vi "test_Create MetaData Channel_error on empty name.vi"(8 "error in (no error)":errorcluster, 11 "TestCase in":refnum<class "Instrument Addon Scripting API Channels Unit Tests.lvclass">) -> (0 "error out":errorcluster, 3 "TestCase out":refnum<class "Instrument Addon Scripting API Channels Unit Tests.lvclass">)   [LabVIEW 2018, in "Instrument Addon Scripting API Channels Unit Tests.lvclass"]
uses:
  Instrument Addon Scripting API Channels Unit Tests.lvclass
  APIs/Scripting API/TypeDefs/Single Channel Format Settings.ctl
  Instrument Addon Scripting API Channels Unit Tests.lvclass/Instrument Addon Scripting API Channels Unit Tests.ctl
  <vilib>/NI Veristand/Custom Device Tools/Custom Device Utility Library/NI VeriStand - Search for Item by Name.vi
  APIs/Scripting API/Channels/Create MetaData Channel - Single Channel - Format.vi
  <vilib>/addons/_JKI Toolkits/VI Tester/TestCase.llb/TestCase.lvclass
  Instrument Addon Scripting API Test Assets/Instrument Addon Scripting API Test Assets.lvclass
  <vilib>/NI Veristand/Custom Device Tools/Custom Device Utility Library/Custom Device Utility Library.lvlib
  APIs/Scripting API/Instrument Addon Scripting API.lvlib
  C:/Program Files (x86)/National Instruments/LabVIEW 2018/vi.lib/addons/_JKI Toolkits/VI Tester/TestCase.llb/TestCase.lvclass
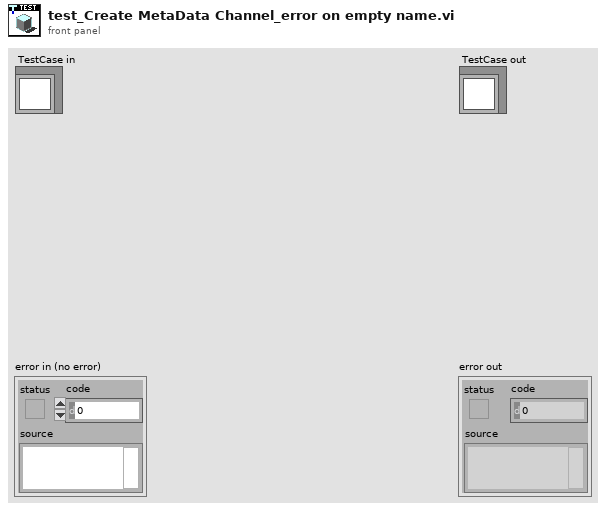
[diagram p1: front panel]
types:
  T1 = typedef "Instrument Addon Scripting API.lvlib/Single Channel Format Settings.ctl" = cluster{"Format String":string, "Default Value":dbl, "Units":string}
  T2 = typedef "Custom Device API.lvlib/Custom Device Item Ref.ctl" = u64
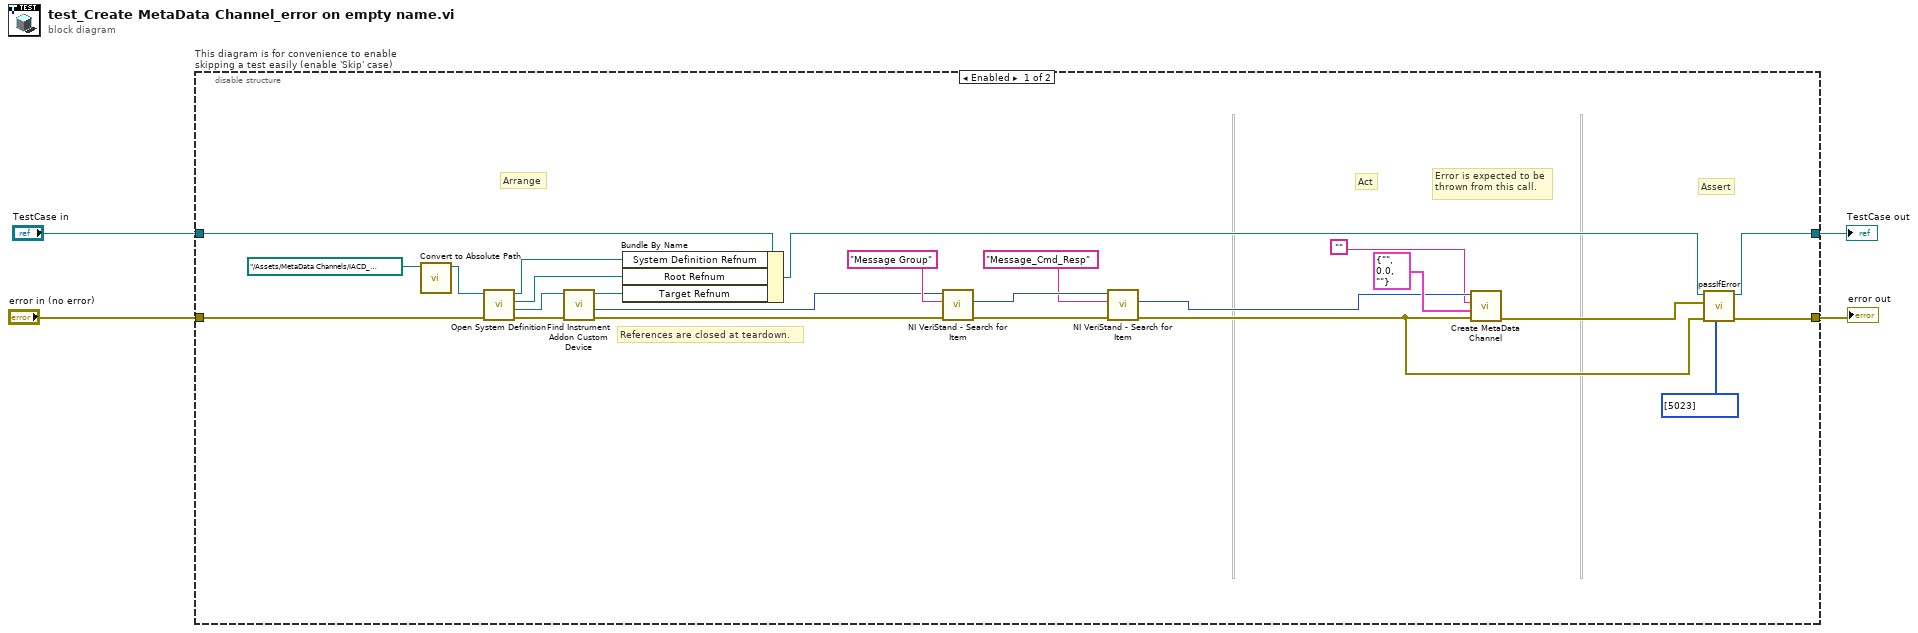
[diagram p0: block diagram]
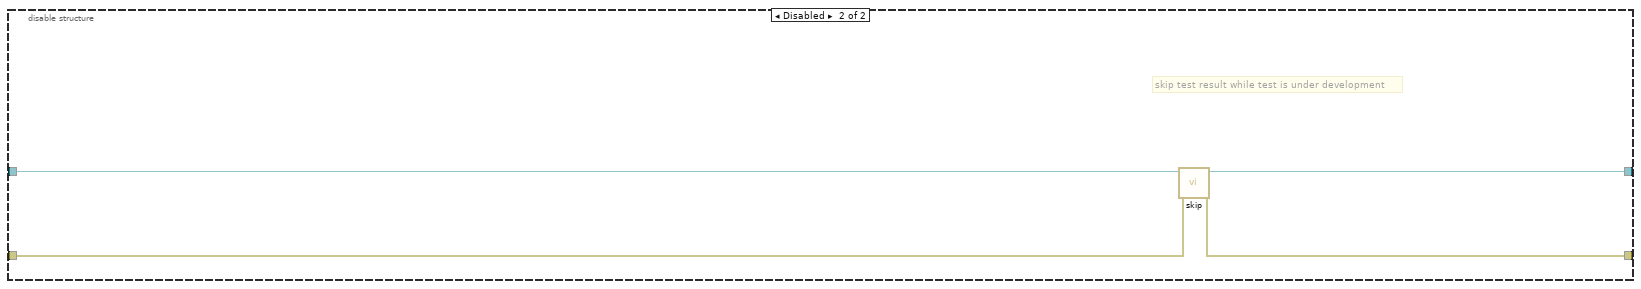
[diagram p2: hidden frame]
diagram:
  n1 = disable-structure "This diagram is for convenience to enable skipping a test easily (enable 'Skip' case)" shown="Enabled" {
    disable-tunnel: "TestCase in" -> [w20 w32]
    disable-tunnel: [w25 w30] -> w1
    disable-tunnel: [w24 w31] -> w3
    disable-tunnel: "error in (no error)" -> [w28 w29]
    frame Enabled {
      # "Error is expected to be\nthrown from this call."
      # "Assert"
      # "References are closed at teardown."
      # "Act"
      # "Arrange"
      n2 = call "Convert to Absolute Path.vi"("System Definition File"=path "../Assets/MetaData Channels/IACD_channels.nivssdf") -> ("Absolute Path"=w5:path)  [unwired: 10 in]
      n3 = call "Open System Definition.vi"("error in (no error)"=w28, "System Definition File"=w5) -> ("error out"=w26:errorcluster, "Target Refnum"=w27:refnum<k24>, "Root Refnum"=w22:refnum<k24>, "System Definition Refnum"=w21:refnum<k24>)  [unwired: 6 in]
      n4 = call "Find Instrument Addon Custom Device.vi"("error in"=w26, "target in"=w27) -> ("error out"=w15:errorcluster, "NodeID"=w14:u64, "target out"=w23:refnum<k24>)  [unwired: 7 in]
      n5 = Bundle By Name(cluster=w20, "System Definition Refnum"=w21, "Root Refnum"=w22, "Target Refnum"=w23) -> (w13:refnum<class "Instrument Addon Scripting API Channels Unit Tests.lvclass">)
      n6 = call-poly <vilib>:"NI VeriStand - Search for Item.vi"("error in"=w15, "Item Name"="Message Group", "Section Ref in"=w14) -> ("error out"=w16:errorcluster, "Item Ref"=w18:T2)  [unwired: 5 in, 2 out]
      n7 = call-poly <vilib>:"NI VeriStand - Search for Item.vi"("error in"=w16, "Item Name"="Message_Cmd_Resp", "Section Ref in"=w18) -> ("error out"=w9:errorcluster, "Item Ref"=w8:T2)  [unwired: 5 in, 2 out]
      n8 = call-poly "Create MetaData Channel.vi"("Error In"=w9, "Settings"=T1 {"Format String"="", "Default Value"=0.0, "Units"=""}, "Name"="", "Message Refnum In"=w8) -> ("Error Out"=w10:errorcluster)  [unwired: 5 in, 2 out]
      n9 = call-dynamic "passIfError.vi"("passing error codes (default = any error code)"=i32[] [5023], "error in (no error)"=w9, "error"=w10, "TestCase in"=w13) -> ("error out"=w24:errorcluster, "TestCase out"=w25:refnum<class "Instrument Addon Scripting API Channels Unit Tests.lvclass">)  [unwired: 6 in]
    }
    frame Disabled {
      # "skip test result while test is under development"
      n10 = call <vilib>:"skip.vi"("error in (no error)"=w29, "TestCase in"=w32) -> ("error out"=w31:errorcluster, "TestCase out"=w30:refnum<class "Instrument Addon Scripting API Channels Unit Tests.lvclass">)  [unwired: 8 in]
    }
  }
  "error out" <- w3
  "TestCase out" <- w1
